vi "Write Instrument Tables.vi"(8 "error in (no error)":errorcluster, 9 "Core Table":variant, 10 "Alias Table":variant, 11 "Multi Instrument Msg in":refnum<class "Multi Instrument Msg.lvclass">) -> (0 "error out":errorcluster, 3 "Multi Instrument Msg out":refnum<class "Multi Instrument Msg.lvclass">)   [LabVIEW 2020, in "Instrument Handler.lvlib" / "Multi Instrument Msg.lvclass"]
doc: "Write the Alias and Core Tables to the private data of the Multi Instrument Msg class."
uses:
  Multi Instrument Msg.lvclass
  Multi Instrument Msg.lvclass/Multi Instrument Msg.ctl
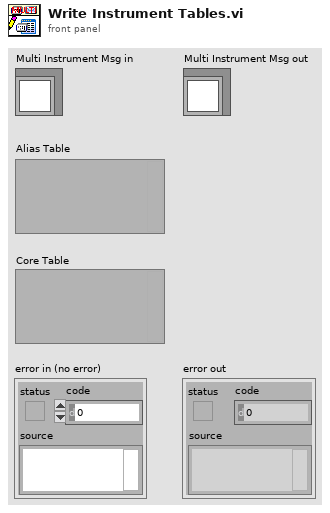
[diagram p1: front panel]
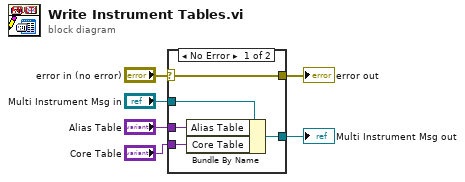
[diagram p0: block diagram]
diagram:
  n1 = case shown="No Error" "error in (no error)" {
    selector: "error in (no error)" -> [w11 w12]
    tunnel: [w11 w12] -> w5
    tunnel: [w9 w13] -> w3
    tunnel: "Multi Instrument Msg in" -> [w10 w13]
    tunnel: "Alias Table" -> [w8 _]
    tunnel: "Core Table" -> [w7 _]
    frame No Error {
      n2 = Bundle By Name(cluster=w10, "Alias Table"=w8, "Core Table"=w7) -> (w9:refnum<class "Multi Instrument Msg.lvclass">)
    }
    frame Error {
    }
  }
  "error out" <- w5
  "Multi Instrument Msg out" <- w3
